vi "Teleop.vi"(10 "Match Info":T1={"Autonomous Elapsed Seconds"=0.0, "TeleOp Elapsed Seconds"=0.0, "Disabled Elapsed Seconds"=0.0, "Visited Autonomous"=FALSE, "Visited TeleOp"=FALSE, "Visited Disabled"=FALSE, "Autonomous Settings"={"Autonomous Style"=enum."Independent", "VI Refnum"=refnum}}, 11 "Call Context":T2) -> ()   [LabVIEW 2019]
doc: "This VI is called for each enabled TeleOp packet received from the DS. It is typically used to read from joysticks and other inputs and update I/O or setpoints for timed control loops. It should complete and return within 20 milliseconds or risk missing DS packets."
uses:
  <vilib>/Rock Robotics/WPI/DriverStation/WPI_DriverStationDerivedRobotMode.ctl
  <vilib>/Rock Robotics/WPI/DriverStation/WPI_DriverStationMatch Info.ctl
  <vilib>/Rock Robotics/WPI/Solenoid/WPI_SolenoidValue.ctl
  <vilib>/Rock Robotics/WPI/Utilities/WPI_GetSetVariantRefNum.vi
  <vilib>/Rock Robotics/Network Tables/NT Write Boolean Array.vi
  <vilib>/Rock Robotics/Network Tables/NT Write Numeric Array.vi
  <vilib>/Rock Robotics/WPI/Solenoid/WPI_SolenoidSetEnum.vi
  <vilib>/Rock Robotics/WPI/Solenoid/WPI_SolenoidGetEnum.vi
  <vilib>/Rock Robotics/WPI/SafetyOutput/WPI_SafetyOutputConfigMenu.ctl
panel:
  in  "Firing":bool
  in  "FireIndex":dbl
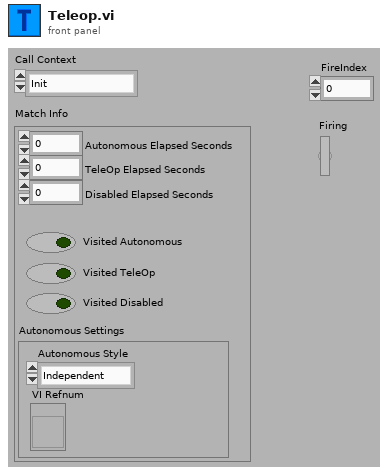
[diagram p1: front panel]
types:
  T1 = typedef "WPI_DriverStationMatch Info.ctl" = cluster{"Autonomous Elapsed Seconds":dbl, "TeleOp Elapsed Seconds":dbl, "Disabled Elapsed Seconds":dbl, "Visited Autonomous":bool, "Visited TeleOp":bool, "Visited Disabled":bool, "Autonomous Settings":cluster{"Autonomous Style":enum16{"Iterative", "Independent"}, "VI Refnum":refnum<vi>}}
  T2 = typedef "WPI_DriverStationDerivedRobotMode.ctl" = enum16{"Init", "Execute", "Stop"}
  T3 = typedef "WPI_JoystickDevRef.ctl" = cluster{"Device":T4}
  T4 = typedef "WPI_JoystickDeviceEnum.ctl" = enum16{"USB 0", "USB 1", "USB 2", "USB 3", "USB 4", "USB 5"}
  T5 = typedef "WPI_SolenoidValue.ctl" = enum16{"Off", "On", "Forward", "Reverse"}
  T6 = typedef "WPI_SolenoidDevRef.ctl" = cluster{"DevStatus":errorcluster, "Pneumatics Control Module":u8, "Forward Solenoid Channel":T7, "Reverse Solenoid Channel":T7}
  T7 = typedef "WPI_SolenoidChannel.ctl" = enum8{"Solenoid 0", "Solenoid 1", "Solenoid 2", "Solenoid 3", "Solenoid 4", "Solenoid 5", "Solenoid 6", "Solenoid 7", "Invalid"}
  T8 = typedef "WPI_SafetyOutputConfigMenu.ctl" = enum16{"Enable", "Disable"}
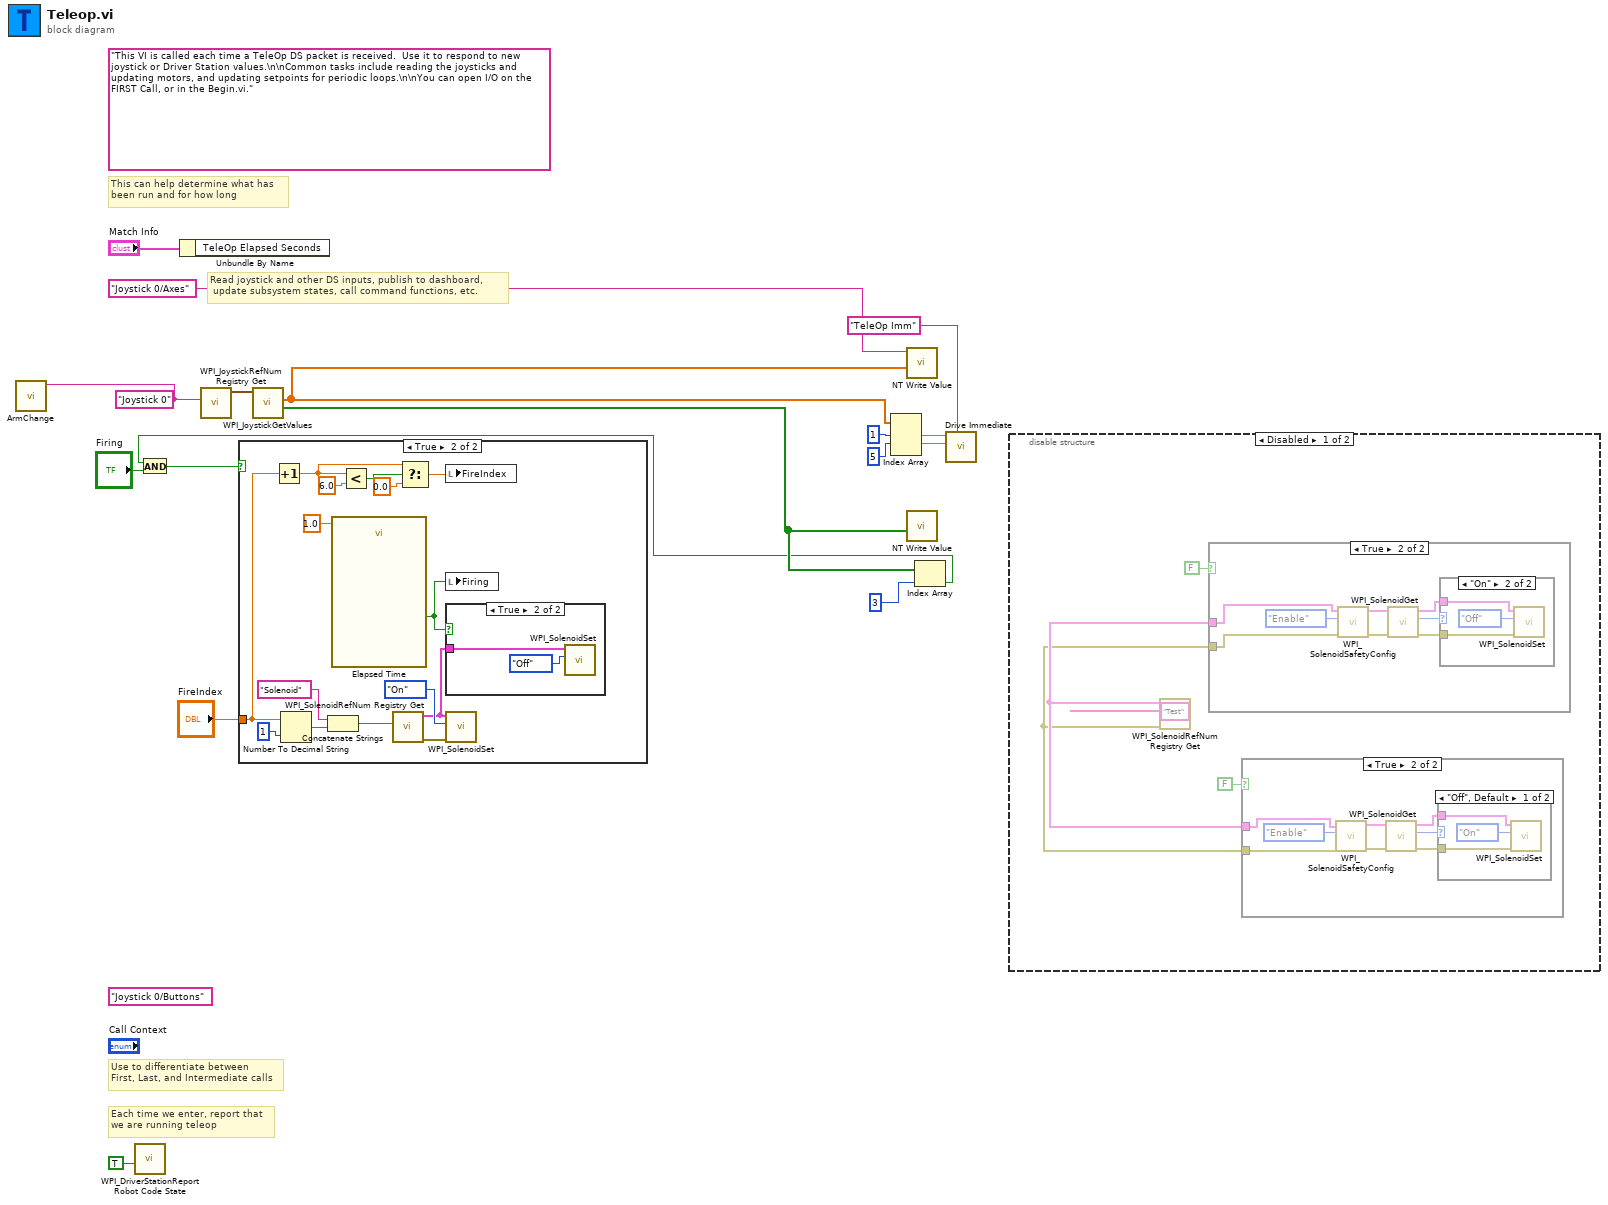
[diagram p0: block diagram]
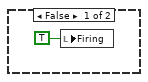
[diagram p7: hidden frame]
diagram:
  (unwired) "Joystick 0/Buttons" ("Name")
  w7 = "Joystick 0" ("refnum name")
  (unwired) "This VI is called each time a TeleOp DS packet is received.  Use it to respond to new joystick or Driver Station values.\n\nCommon tasks include reading the joysticks and updating motors, and updating setpoints for periodic loops.\n\nYou can open I/O on the FIRST Call, or in the Begin.vi."
  # "Read joystick and other DS inputs, publish to dashboard,\n update subsystem states, call command functions, etc."
  # "Each time we enter, report that\nwe are running teleop"
  # "Use to differentiate between\nFirst, Last, and Intermediate calls"
  # "This can help determine what has\nbeen run and for how long"
  n1 = call "ArmChange.vi"("refnum name"=w7) -> ()  [unwired: 11 in]
  n2 = call <vilib>:"WPI_DriverStationReport Robot Code State.vi"("TeleOp"=TRUE ("Autonomous")) -> ()  [unwired: 10 in, 1 out]
  n3 = Unbundle By Name("Match Info") -> ()  [unwired: 1 out]
  n4 = call <vilib>:"WPI_JoystickRefNum Registry Get.vi"("refnum name"=w7) -> ("JoystickDevRef"=w15:T3)  [unwired: 1 in, 9 out]
  n5 = call <vilib>:"WPI_JoystickGetValues.vi"("JoystickDevRef"=w15) -> ("Buttons"=w6:bool[], "Axes"=w10:dbl[])  [unwired: 6 in, 3 out]
  n6 = Index Array(array=w10, index #1=1 ("index"), index #2=5 ("index")) -> (element #1=w12:dbl, element #2=w13:dbl)  [unwired: 1 in, 1 out]
  n7 = call-poly <vilib>:"NT Write Value.vi"("Numeric Array"=w10, "Name"="Joystick 0/Axes") -> ()  [unwired: 9 in, 1 out]
  n8 = call-poly <vilib>:"NT Write Value.vi"("Boolean Array"=w6) -> ()  [unwired: 10 in, 1 out]
  n9 = Index Array(array=w6, index=3) -> (element=w3:bool)
  n10 = And(x=w3, y="Firing") -> (x .and. y?=w1:bool)
  n11 = case shown="True" w1 {
    tunnel: "FireIndex" -> [_ w20]
    frame False {
      n12 = local write "Firing"(TRUE) -> ()
    }
    frame True {
      n13 = Increment(x=w20) -> (x+1=w24:dbl)
      n14 = Number To Decimal String(number=w20, width (-)=i16 1) -> (decimal integer string=w28:string)
      n15 = Concatenate Strings("Solenoid" ("string"), w28) -> (w30:string)
      n16 = call "Elapsed Time"("Time Target (s)"=1.0) -> ("Time has Elapsed"=w19:bool)  [unwired: 11 in, 7 out]
      n17 = Less?(x=w24, y=6.0) -> (x < y?=w25:bool)
      n18 = call <vilib>:"WPI_SolenoidRefNum Registry Get.vi"("refnum name"=w30) -> ("error out"=w32:errorcluster, "SolenoidDevRef"=w31:T6)  [unwired: 9 in]
      n19 = Select(t=w24, s=w25, f=0.0) -> (s? t:f=w22:dbl)
      n20 = local write "FireIndex"(w22) -> ()
      n21 = local write "Firing"(w19) -> ()
      n22 = case shown="True" w19 {
        tunnel: w31 -> [_ w34]
        frame False {
        }
        frame True {
          n23 = call-poly <vilib>:"WPI_SolenoidSet.vi"("Value"=WPI_SolenoidValue."Off", "SolenoidDevRef"=w34) -> ()  [unwired: 8 in, 2 out]
        }
      }
      n24 = call-poly <vilib>:"WPI_SolenoidSet.vi"("error in (no error)"=w32, "Value"=WPI_SolenoidValue."On", "SolenoidDevRef"=w31) -> ()  [unwired: 7 in, 2 out]
    }
  }
  n25 = call "Drive Immediate.vi"("Description"="TeleOp Imm", "Right Setpoint"=w13, "Left Setpoint"=w12) -> ()  [unwired: 8 in, 1 out]
  n26 = disable-structure shown="Disabled" {
    frame Disabled {
      n27 = call <vilib>:"WPI_SolenoidRefNum Registry Get.vi"("refnum name"="Test") -> ("error out"=w38:errorcluster, "SolenoidDevRef"=w39:T6)  [unwired: 9 in]
      n28 = case shown="True" FALSE {
        tunnel: w38 -> [_ w56]
        tunnel: w39 -> [_ w57]
        frame False {
        }
        frame True {
          n29 = call <vilib>:"WPI_SolenoidSafetyConfig.vi"("error in (no error)"=w56, "mode"=WPI_SafetyOutputConfigMenu."Enable", "SolenoidDevRef"=w57) -> ("error out"=w54:errorcluster, "SolenoidDevRef"=w55:T6)  [unwired: 7 in]
          n30 = call-poly <vilib>:"WPI_SolenoidGet.vi"("error in (no error)"=w54, "SolenoidDevRef"=w55) -> ("error out"=w52:errorcluster, "Value"=w59:T5, "SolenoidDevRef"=w53:T6)  [unwired: 7 in]
          n31 = case shown="\"On\"" w59 {
            tunnel: w53 -> [_ w61]
            tunnel: w52 -> [_ w60]
            frame "Off", Default {
            }
            frame "On" {
              n32 = call-poly <vilib>:"WPI_SolenoidSet.vi"("error in (no error)"=w60, "Value"=WPI_SolenoidValue."Off", "SolenoidDevRef"=w61) -> ()  [unwired: 7 in, 2 out]
            }
          }
        }
      }
      n33 = case shown="True" FALSE {
        tunnel: w38 -> [_ w43]
        tunnel: w39 -> [_ w44]
        frame False {
        }
        frame True {
          n34 = call <vilib>:"WPI_SolenoidSafetyConfig.vi"("error in (no error)"=w43, "mode"=WPI_SafetyOutputConfigMenu."Enable", "SolenoidDevRef"=w44) -> ("error out"=w41:errorcluster, "SolenoidDevRef"=w42:T6)  [unwired: 7 in]
          n35 = call-poly <vilib>:"WPI_SolenoidGet.vi"("error in (no error)"=w41, "SolenoidDevRef"=w42) -> ("error out"=w45:errorcluster, "Value"=w48:T5, "SolenoidDevRef"=w46:T6)  [unwired: 7 in]
          n36 = case shown="\"Off\", Default" w48 {
            tunnel: w46 -> [w50 _]
            tunnel: w45 -> [w49 _]
            frame "Off", Default {
              n37 = call-poly <vilib>:"WPI_SolenoidSet.vi"("error in (no error)"=w49, "Value"=WPI_SolenoidValue."On", "SolenoidDevRef"=w50) -> ()  [unwired: 7 in, 2 out]
            }
            frame "On" {
            }
          }
        }
      }
    }
    frame Enabled {
    }
  }
